vi "Test_HelloWorld.vi"() -> (0 "Array of Error Description":T1)   [LabVIEW 2025]
uses:
  gRPC_ATS/TestUtility/utility.llb/array of error description.ctl
  gRPC_ATS/TestUtility/utility.llb/error description.ctl
  gRPC_ATS/TestUtility/utility.llb/error type.ctl
  examples/helloworld/helloworld_client/RPC Messages/helloworld_HelloRequest.ctl
  examples/helloworld/helloworld_client/RPC Messages/helloworld_HelloReply.ctl
  examples/helloworld/helloworld_client/helloworld_client.lvlib
panel:
  out "Pass":bool
  in  "Client VI Path":path=path "../../examples/helloworld/helloworld_client/Run greeter_client.vi"
  in  "Server VI path":path=path "../../examples/helloworld/helloworld_server/Run greeter_server.vi"
  in  "error in (no error)":errorcluster
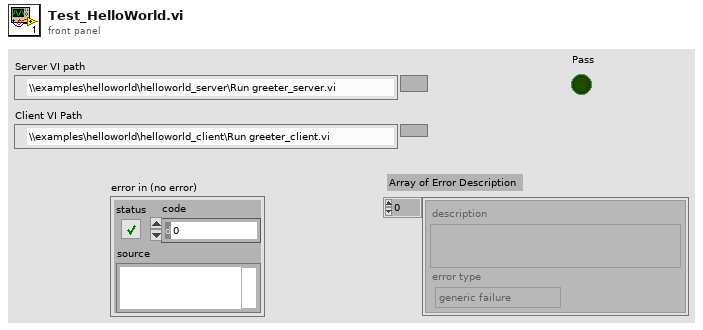
[diagram p1: front panel]
types:
  T1 = typedef "array of error description.ctl" = T2[]
  T2 = typedef "error description.ctl" = cluster{"description":string, "error type":T3}
  T3 = typedef "error type.ctl" = enum32{"generic failure", "boundary case", "precision", "expected error"}
  T4 = typedef "helloworld_client.lvlib/helloworld_HelloReply.ctl" = cluster{"message":string}
  T5 = typedef "helloworld_client.lvlib/helloworld_HelloRequest.ctl" = cluster{"name":string}
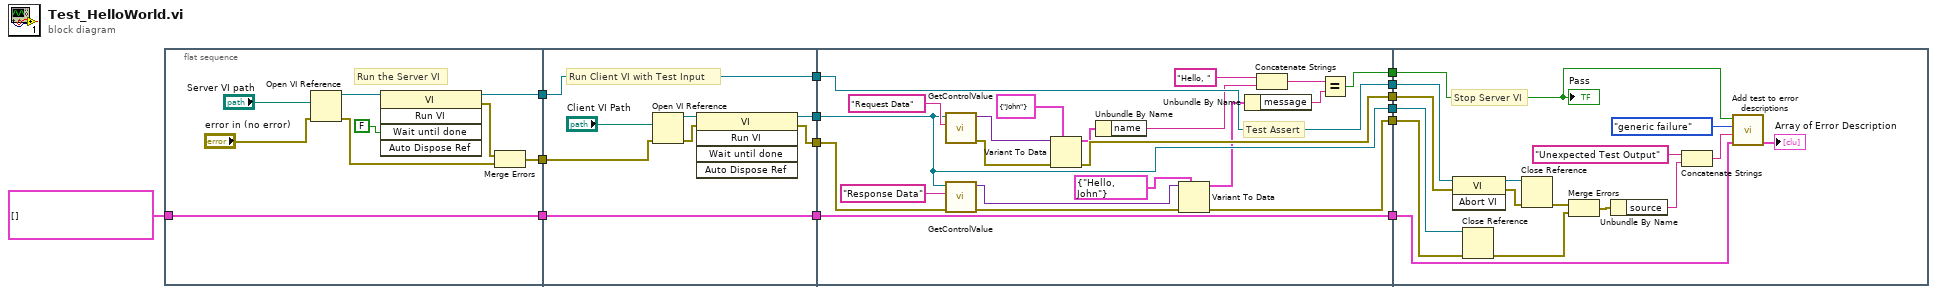
[diagram p0: block diagram]
diagram:
  n1 = flat-sequence {
    tunnel: T1 [] ("error descriptions in") -> [w19]
    tunnel: [w19] -> w14
    tunnel: [w18] -> w13
    tunnel: [w15] -> w12
    tunnel: w14 -> [w30]
    tunnel: [w30] -> w11
    tunnel: [w29] -> w10
    tunnel: w13 -> [w29]
    tunnel: w12 -> [w28]
    tunnel: [w25] -> w5
    tunnel: [w24] -> w4
    tunnel: w11 -> [w51]
    tunnel: [w51] -> w9
    tunnel: [w38] -> w8
    tunnel: w10 -> [w38]
    tunnel: [w52] -> w6
    tunnel: w5 -> [w48]
    tunnel: w4 -> [w41]
    tunnel: [w41] -> w3
    tunnel: [w40] -> w2
    tunnel: [w39] -> w1
    tunnel: w9 -> [w63]
    tunnel: w8 -> [w60]
    tunnel: w6 -> [w59]
    tunnel: w3 -> [w55]
    tunnel: w2 -> [w54]
    tunnel: w1 -> [w53]
    frame #0 {
      # "Run the Server VI"
      n2 = Open VI Reference(vi path="Server VI path", error in (no error)="error in (no error)") -> (vi reference=w21:refnum<vi>, error out=w17:errorcluster)  [unwired: 4 in]
      n3 = invoke class="VI" method="Run VI"(reference=w21, "Wait until done"=FALSE ("Wait Until Done")) -> (reference out=w18:refnum<vi>, error out=w16:errorcluster)  [unwired: 3 in, 3 out]
      n4 = Merge Errors(w16, w17) -> (w15:errorcluster)
    }
    frame #1 {
      # "Run Client VI with Test Input"
      n5 = Open VI Reference(vi path="Client VI Path", error in (no error)=w28) -> (vi reference=w26:refnum<vi>, error out=w27:errorcluster)  [unwired: 4 in]
      n6 = invoke class="VI" method="Run VI"(reference=w26, error in=w27) -> (reference out=w24:refnum<vi>, error out=w25:errorcluster)  [unwired: 3 in, 3 out]
    }
    frame #2 {
      # "Test Assert"
      n7 = call "GetControlValue.vi"("Control Label"="Request Data", "VI Reference"=w41) -> ("error out"=w43:errorcluster, "Value"=w42:variant)  [unwired: 8 in]
      n8 = call "GetControlValue.vi"("error in (no error)"=w48, "Control Label"="Response Data", "VI Reference"=w41) -> ("error out"=w46:errorcluster, "Value"=w45:variant)  [unwired: 7 in]
      n9 = Variant To Data(error in=w43, type=T5 {"name"="John"} ("Request Data"), Variant=w42) -> (data=w36:T5, error out=w39:errorcluster)
      n10 = Unbundle By Name(w36) -> ("name"=w35:string)
      n11 = Variant To Data(error in=w46, type=T4 {"message"="Hello, John"} ("Response Data"), Variant=w45) -> (data=w33:T4, error out=w40:errorcluster)
      n12 = Unbundle By Name(w33) -> ("message"=w32:string)
      n13 = Concatenate Strings("Hello, " ("string"), w35) -> (w49:string)
      n14 = Equal?(x=w49, y=w32) -> (x = y?=w52:bool)
    }
    frame #3 {
      # "Stop Server VI"
      n15 = invoke class="VI" method="Abort VI"(reference=w60, error in=w53) -> (reference out=w61:refnum<vi>, error out=w62:errorcluster)  [unwired: 1 in, 1 out]
      n16 = Close Reference(reference=w55, error in (no error)=w54) -> (error out=w57:errorcluster)
      n17 = Close Reference(reference=w61, error in (no error)=w62) -> (error out=w58:errorcluster)
      n18 = Merge Errors(w58, w57) -> (w56:errorcluster)
      n19 = Unbundle By Name(w56) -> ("source"=w65:string)
      n20 = Concatenate Strings("Unexpected Test Output" ("string"), w65) -> (w66:string)
      n21 = call "Add test to error descriptions.vi"("error descriptions in"=w63, "error string"=w66, "error type"=error_type."generic failure", "pass"=w59) -> ("error description out"=→"Array of Error Description":T1)  [unwired: 3 in]
      "Pass" <- w59
    }
  }
